vi "程序退出.vi"(6 "error in (no error)":errorcluster, 9 "仪器实例 in":T1) -> (0 "error out":errorcluster)   [LabVIEW 2020]
uses:
  F:/F020/S7_1200 control/HslCommunication.dll
  S7_1200 control/HslCommunication.dll
  S7_1200 control/S7_1200 WriteBools.vi
  S7_1200 control/S7_1200 control.lvlib
  <instrlib>/IT6300/IT6300.lvlib
  <instrlib>/Keithley 27XX/Keithley 27XX.lvlib
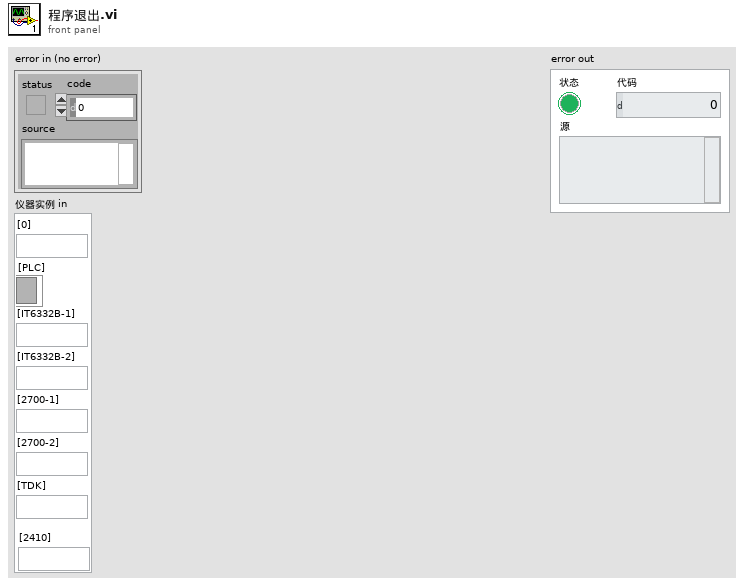
[diagram p1: front panel]
types:
  T1 = typedef "仪器实例.ctl" = cluster{"[0]":string, "[PLC]":refnum<k24>, "[IT6332B-1]":string, "[IT6332B-2]":string, "[2700-1]":string, "[2700-2]":string, "[TDK]":string, "[2410]":string}
  T2 = cluster{"Channel1":bool, "Channel2":bool, "Channel3":bool}
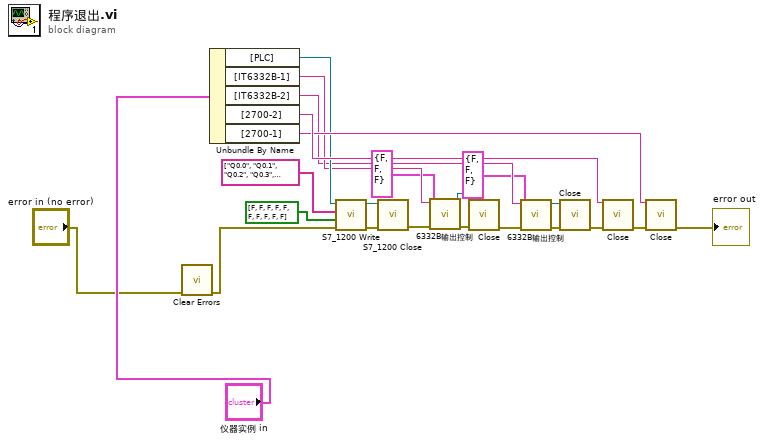
[diagram p0: block diagram]
diagram:
  n1 = call <vilib>:"Clear Errors.vi"("error in (no error)"="error in (no error)") -> ("error out"=w1:errorcluster)  [unwired: 5 in, 1 out]
  n2 = Unbundle By Name("仪器实例 in") -> ("[PLC]"=w15:refnum<k24>, "[IT6332B-1]"=w12:string, "[IT6332B-2]"=w7:string, "[2700-2]"=w20:string, "[2700-1]"=w19:string)
  n3 = call-poly "S7_1200 Write.vi"("错误输入（无错误）"=w1, "values"=bool[] [FALSE, FALSE, FALSE, FALSE, FALSE, FALSE, FALSE, FALSE, FALSE, FALSE], "addresses"=string[] ["Q0.0", "Q0.1", "Q0.2", "Q0.3", "Q0.4", "Q0.5", "Q0.6", "Q0.7", "Q1.0", "Q1.1"], "引用"=w15) -> ("错误输出"=w13:errorcluster, "引用输出"=w14:refnum<k24>)  [unwired: 2 in]
  n4 = call "S7_1200 Close.vi"("错误输入（无错误）"=w13, "引用输出"=w14) -> ("错误输出"=w11:errorcluster)  [unwired: 5 in]
  n5 = call "6332B输出控制.vi"("错误输入"=w11, "Choose Channel"=T2 {"Channel1"=FALSE, "Channel2"=FALSE, "Channel3"=FALSE}, "VISA资源名称"=w12) -> ("错误输出"=w10:errorcluster, "VISA资源名称输出"=w3:refnum<visa-resource-name>)  [unwired: 7 in]
  n6 = call <instrlib>:"Close.vi"("error in (no error)"=w10, "VISA resource name"=w3) -> ("error out"=w5:errorcluster)  [unwired: 9 in]
  n7 = call "6332B输出控制.vi"("错误输入"=w5, "Choose Channel"=T2 {"Channel1"=FALSE, "Channel2"=FALSE, "Channel3"=FALSE}, "VISA资源名称"=w7) -> ("错误输出"=w9:errorcluster, "VISA资源名称输出"=w8:refnum<visa-resource-name>)  [unwired: 7 in]
  n8 = call <instrlib>:"Close.vi"("error in (no error)"=w9, "VISA resource name"=w8) -> ("error out"=w21:errorcluster)  [unwired: 9 in]
  n9 = call <instrlib>:"Close.vi"("VISA resource name"=w20, "error in (no error)"=w21) -> ("error out"=w18:errorcluster)  [unwired: 13 in]
  n10 = call <instrlib>:"Close.vi"("VISA resource name"=w19, "error in (no error)"=w18) -> ("error out"=→"error out":errorcluster)  [unwired: 13 in]
